vi "1 Ball Center Half Hot.vi"(1 "Run?":bool) -> (0 "Done?":bool)   [LabVIEW 2013]
uses:
  Globals/Homes.vi
  Globals/Useful Values.vi
panel:
  out "Sum":dbl
  out "Vision Decided":dbl
  out "Ready for Vision?":bool
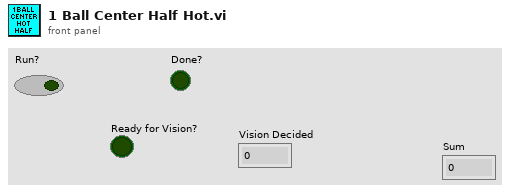
[diagram p1: front panel]
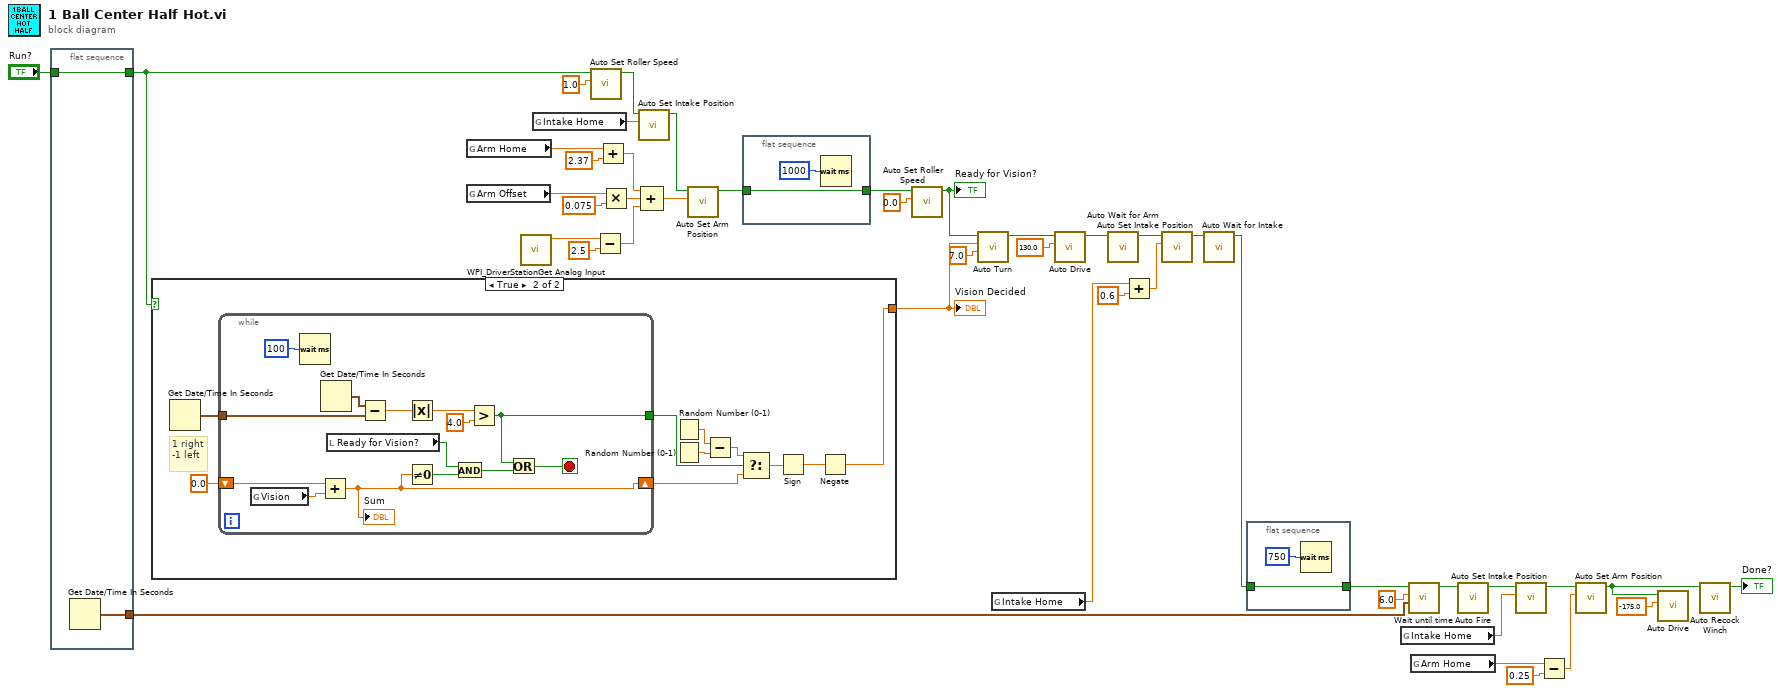
[diagram p0: block diagram]
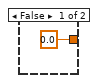
[diagram p2: hidden frame]
diagram:
  n1 = flat-sequence {
    tunnel: [w46] -> w14
    tunnel: [w45] -> w16
    tunnel: "Run?" -> [w45]
    frame #0 {
      n2 = Get Date/Time In Seconds() -> (seconds since 1Jan1904=w46:timestamp)
    }
  }
  n3 = case shown="True" w16 {
    tunnel: [0.0 w48] -> w21
    frame False {
    }
    frame True {
      # "1 right\n-1 left"
      n4 = Get Date/Time In Seconds() -> (seconds since 1Jan1904=w55:timestamp)
      n5 = while {
        shift-right: [w67] -> w50
        shift-left: 0.0 -> [w70]
        tunnel: w55 -> [w65]
        tunnel: [w58] -> w51
        stop <- w60 stop-if-true
        n6 = global read "Useful Values.vi" "Vision"() -> (w71:dbl)
        n7 = Wait (ms)(milliseconds to wait=u32 100) -> ()  [unwired: 1 out]
        n8 = Add(x=w70, y=w71) -> (x+y=w67:dbl)
        "Sum" <- w67
        n9 = Get Date/Time In Seconds() -> (seconds since 1Jan1904=w64:timestamp)
        n10 = local read "Ready for Vision?"() -> (w68:bool)
        n11 = Subtract(x=w64, y=w65) -> (x-y=w63:dbl)
        n12 = Absolute Value(x=w63) -> (abs(x)=w62:dbl)
        n13 = Not Equal To 0?(x=w67) -> (x != 0?=w66:bool)
        n14 = And(x=w68, y=w66) -> (x .and. y?=w59:bool)
        n15 = Greater?(x=w62, y=4.0) -> (0:w58:bool)
        n16 = Or(x=w58, y=w59) -> (x .or. y?=w60:bool)
      }
      n17 = Random Number (0-1)() -> (number: 0 to 1=w52:dbl)
      n18 = Random Number (0-1)() -> (number: 0 to 1=w53:dbl)
      n19 = Subtract(x=w52, y=w53) -> (x-y=w54:dbl)
      n20 = Select(t=w54, s=w51, f=w50) -> (s? t:f=w49:dbl)
      n21 = Sign(1:w49) -> (0:w56:dbl)
      n22 = Negate(x=w56) -> (-x=w48:dbl)
    }
  }
  "Vision Decided" <- w21
  n23 = global read "Homes.vi" "Arm Home"() -> (w9:dbl)
  n24 = global read "Useful Values.vi" "Arm Offset"() -> (w6:dbl)
  n25 = call <vilib>:"WPI_DriverStationGet Analog Input.vi"() -> ("Analog 1 (V)"=w3:dbl)  [unwired: 8 in, 3 out]
  n26 = global read "Homes.vi" "Intake Home"() -> (w38:dbl)
  n27 = call "Auto Set Roller Speed.vi"("Value"=1.0, "Run?"=w16) -> ("Done"=w29:bool)  [unwired: 9 in]
  n28 = Subtract(x=w3, y=2.5) -> (x-y=w2:dbl)
  n29 = Add(x=w9, y=2.37) -> (x+y=w5:dbl)
  n30 = Multiply(x=w6, y=0.075) -> (x*y=w8:dbl)
  n31 = call "Auto Set Intake Position.vi"("Intake Position"=w38, "Run?"=w29) -> ("Done"=w19:bool)  [unwired: 9 in]
  n32 = Compound Arithmetic op=ADD(w5, w8, w2) -> (w1:dbl)
  n33 = call "Auto Set Arm Position.vi"("Arm Position"=w1, "Run?"=w19) -> ("Done"=w20:bool)  [unwired: 9 in]
  n34 = flat-sequence {
    tunnel: w20 -> [w73]
    tunnel: [w73] -> w27
    frame #0 {
      n35 = Wait (ms)(milliseconds to wait=u32 1000) -> ()  [unwired: 1 out]
    }
  }
  n36 = call "Auto Set Roller Speed.vi"("Value"=0.0, "Run?"=w27) -> ("Done"=w22:bool)  [unwired: 9 in]
  "Ready for Vision?" <- w22
  n37 = call "Auto Turn.vi"("Turn Amount"=7.0, "+/-?"=w21, "Run?"=w22) -> ("Done"=w26:bool)  [unwired: 8 in]
  n38 = global read "Homes.vi" "Intake Home"() -> (w39:dbl)
  n39 = call "Auto Drive.vi"("Amount"=130.0, "Run?"=w26) -> ("Done"=w24:bool)  [unwired: 9 in]
  n40 = call "Auto Wait for Arm.vi"("Run?"=w24) -> ("Done"=w25:bool)  [unwired: 10 in]
  n41 = Add(x=w39, y=0.6) -> (x+y=w43:dbl)
  n42 = call "Auto Set Intake Position.vi"("Intake Position"=w43, "Run?"=w25) -> ("Done"=w28:bool)  [unwired: 9 in]
  n43 = call "Auto Wait for Intake.vi"("Run?"=w28) -> ("Done"=w32:bool)  [unwired: 10 in]
  n44 = flat-sequence {
    tunnel: w32 -> [w74]
    tunnel: [w74] -> w12
    frame #0 {
      n45 = Wait (ms)(milliseconds to wait=u32 750) -> ()  [unwired: 1 out]
    }
  }
  n46 = global read "Homes.vi" "Intake Home"() -> (w37:dbl)
  n47 = call "Wait until time.vi"("Initial Time"=w14, "Time to wait for"=6.0, "Run?"=w12) -> ("Done"=w11:bool)  [unwired: 8 in]
  n48 = global read "Homes.vi" "Arm Home"() -> (w34:dbl)
  n49 = call "Auto Fire.vi"("Run?"=w11) -> ("Done"=w42:bool)  [unwired: 10 in]
  n50 = call "Auto Set Intake Position.vi"("Intake Position"=w37, "Run?"=w42) -> ("Done"=w41:bool)  [unwired: 9 in]
  n51 = Subtract(x=w34, y=0.25) -> (x-y=w35:dbl)
  n52 = call "Auto Set Arm Position.vi"("Arm Position"=w35, "Run?"=w41) -> ("Done"=w18:bool)  [unwired: 9 in]
  n53 = call "Auto Drive.vi"("Amount"=-175.0, "Run?"=w18) -> ()  [unwired: 9 in, 1 out]
  n54 = call "Auto Recock Winch.vi"("Run?"=w18) -> ("Done"=→"Done?":bool)  [unwired: 10 in]
